vi "HXG2air-glyClusterFGV.vi"(7 "AirGlyCtrl":T4, 8 "error in (no error)":errorcluster, 10 "Gly Cluster":T3 {"Liq TEMP %" min=0.0 max=100.0 step=1.0 format="%#.1f"; "Liq FLOW %" min=0.0 max=100.0 step=1.0 format="%#.1f"; "TLiq °F" min=40.0 max=180.0 step=1.0 format="%#.1f"; "Mdot lbm/hr" min=0.0 max=1000.0 step=1.0 format="%#.1f"}, 11 "Air Cluster":T2 {"Air TEMP %" min=0.0 max=100.0 step=1.0 format="%#.1f"; "Air FLOW %" min=0.0 max=100.0 step=1.0 format="%#.1f"; "Tair  °F" min=-5.0 max=100.0 step=1.0 format="%#.1f"; "CFMs" min=0.0 max=200.0 step=1.0 format="%#.1f"}) -> (0 "error out":errorcluster, 3 "AIR-GLY Cluster":T1 {"Liq Cluster"."Liq TEMP %" min=0.0 max=100.0 step=1.0 format="%#.1f"; "Liq Cluster"."Liq FLOW %" min=0.0 max=100.0 step=1.0 format="%#.1f"; "Liq Cluster"."TLiq °F" min=40.0 max=180.0 step=1.0 format="%#.1f"; "Liq Cluster"."Mdot lbm/hr" min=0.0 max=1000.0 step=1.0 format="%#.1f"; "Air Cluster"."Air TEMP %" min=0.0 max=100.0 step=1.0 format="%#.1f"; "Air Cluster"."Air FLOW %" min=0.0 max=100.0 step=1.0 format="%#.1f"; "Air Cluster"."Tair  °F" min=-5.0 max=100.0 step=1.0 format="%#.1f"; "Air Cluster"."CFMs" min=0.0 max=200.0 step=1.0 format="%#.1f"})   [LabVIEW 2012]
uses:
  Controls/UI/HXG2_UI_ControlSetGly.ctl
  Controls/UI/HXG2_UI_ControlSetAir.ctl
  HXG2airglyCluster.ctl
  Controls/HXG2_AirGly-Cluster.ctl
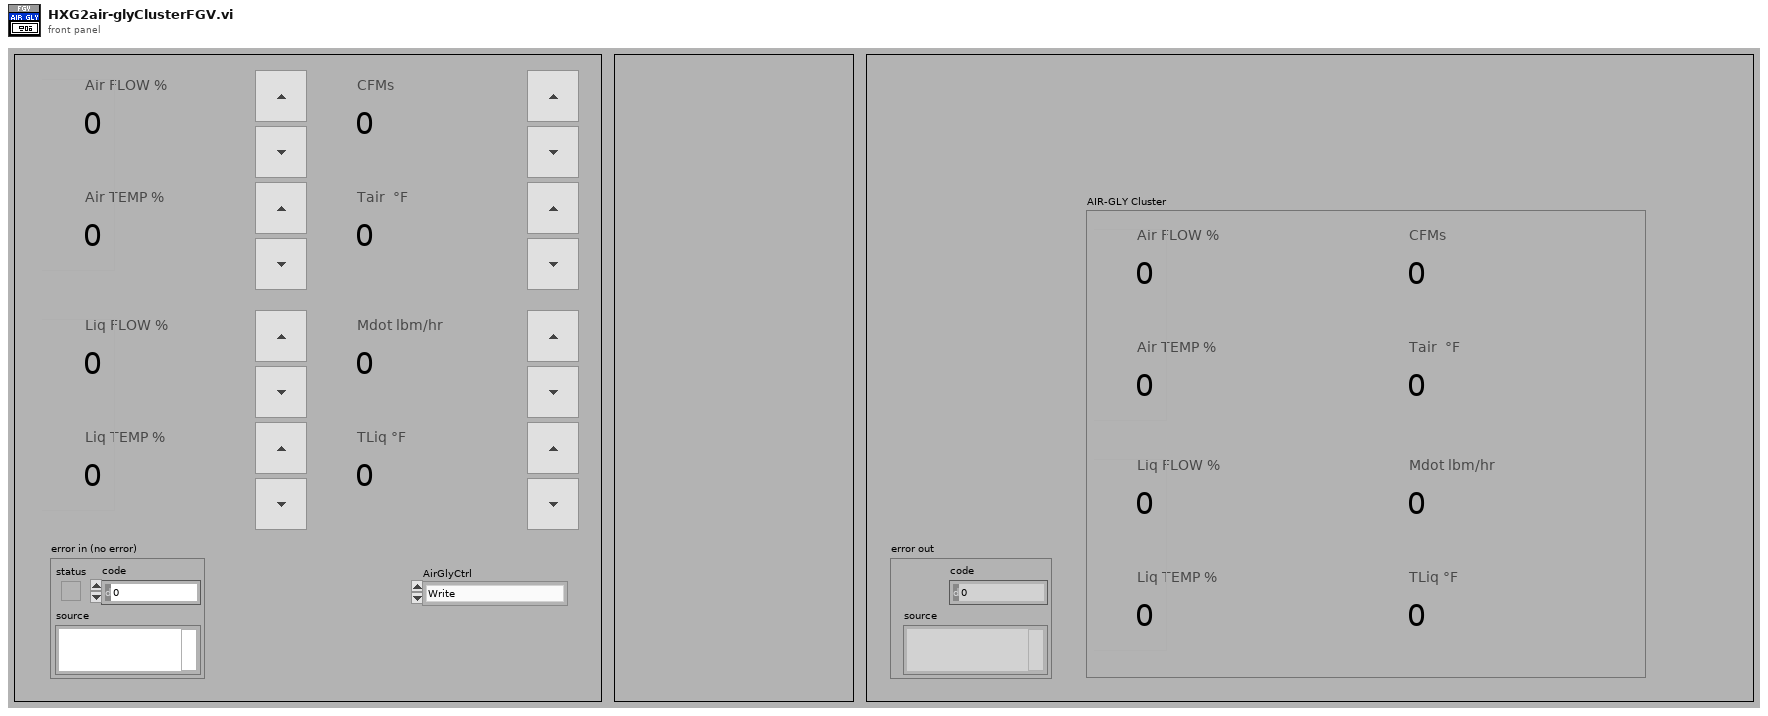
[diagram p1: front panel]
types:
  T1 = typedef "HXG2_AirGly-Cluster.ctl" = cluster{"Air Cluster":T2, "Liq Cluster":T3}
  T2 = typedef "HXG2_UI_ControlSetAir.ctl" = cluster{"Air FLOW %":dbl, "Air TEMP % ":dbl, "CFMs":dbl, "Tair  °F":dbl}
  T3 = typedef "HXG2_UI_ControlSetGly.ctl" = cluster{"Liq FLOW %":dbl, "Liq TEMP % ":dbl, "Mdot lbm/hr":dbl, "TLiq °F":dbl}
  T4 = typedef "HXG2airglyCluster.ctl" = enum16{"Write", "Pass"}
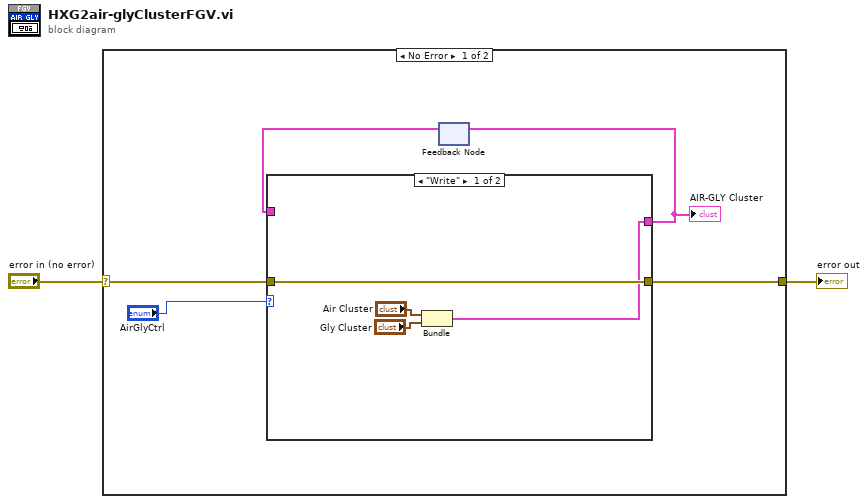
[diagram p0: block diagram]
diagram:
  n1 = case shown="No Error" "error in (no error)" {
    selector: "error in (no error)" -> [w7 w14]
    tunnel: [w6 w14] -> w1
    frame No Error {
      n2 = feedback #1() -> (w5:cluster{"Air Cluster":T2, "Gly Cluster":T3})  [unwired: 1 in]
      n3 = case shown="\"Write\"" "AirGlyCtrl" {
        tunnel: w7 -> [w11 w12]
        tunnel: [w11 w12] -> w6
        tunnel: [w8 w13] -> w3
        tunnel: w5 -> [_ w13]
        frame "Write" {
          n4 = Bundle("Air Cluster"="Air Cluster", "Gly Cluster"="Gly Cluster") -> (w8:cluster{"Air Cluster":T2, "Gly Cluster":T3})  [unwired: 1 in]
        }
        frame "Pass" {
        }
      }
      "AIR-GLY Cluster" <- w3
      n5 = feedback-in #1(w3) -> ()
    }
    frame Error {
    }
  }
  "error out" <- w1
